vi "flipAndAverageBidirectional.vi"(2 "Depth":dbl[][](graph), 3 "Scan in":refnum<class "Scan.lvclass">) -> (0 "Depth out":dbl[][](graph))   [LabVIEW 2017]
uses:
  classes/Scans/Scan.lvclass
  classes/Scans/Scan.lvclass/Scan.ctl
  classes/Scans/Read A scans.vi
  classes/Scans/Read Total A-scans per frame.vi
  classes/Scans/Read Bidirectional.vi
panel:
  out "size(s) 3":i32[](array[numeric])
  out "size(s) 2":i32[](array[numeric])
  out "size(s)":i32[](array[numeric])
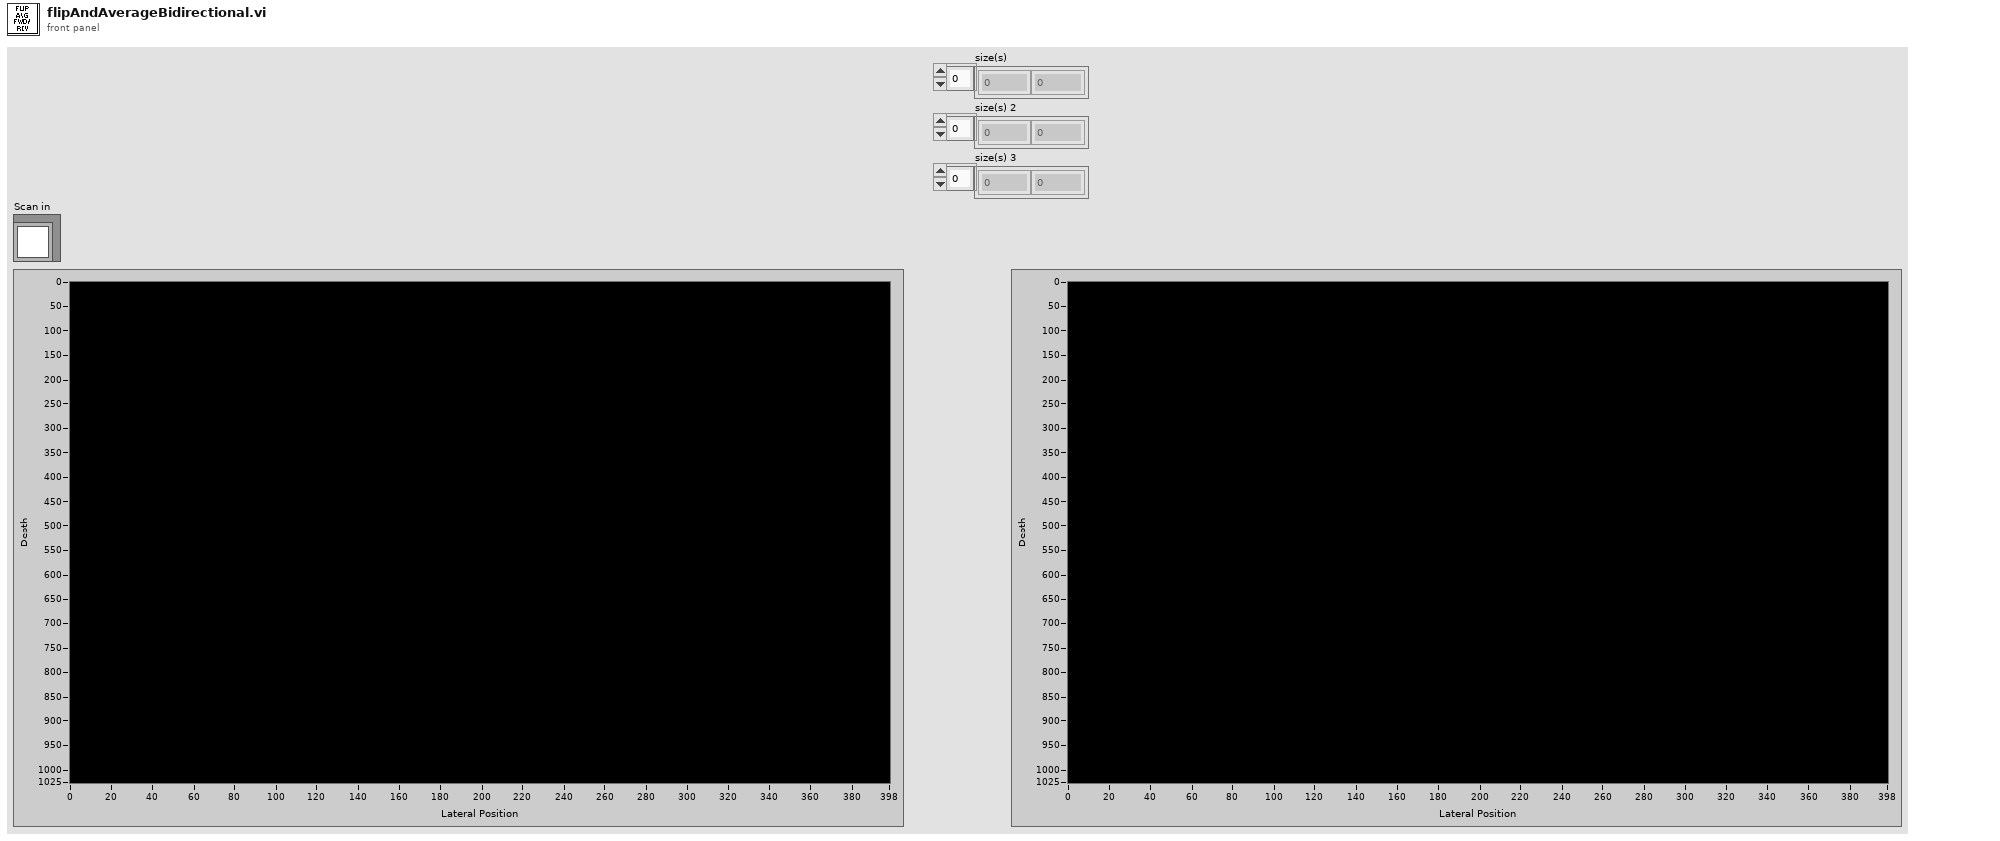
[diagram p1: front panel]
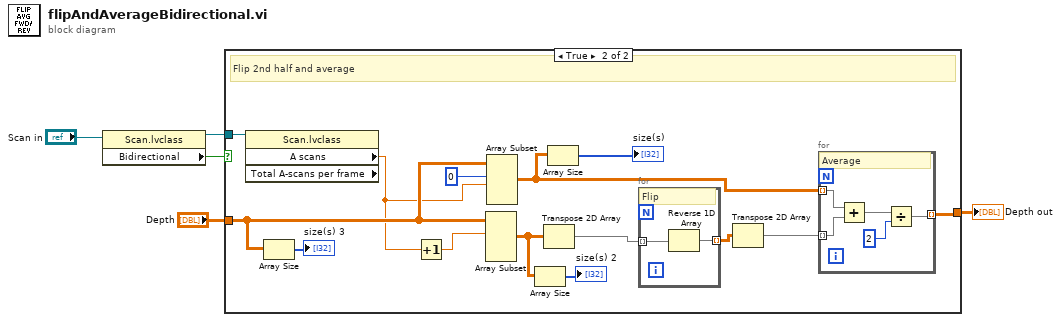
[diagram p0: block diagram]
diagram:
  n1 = property class="Scan.lvclass"(reference="Scan in") -> (reference out=w1:refnum<class "Scan.lvclass">, "Bidirectional"=w4:bool)  [unwired: 1 in, 1 out]
  n2 = case shown="True" w4 {
    tunnel: [w6 w17] -> w2
    tunnel: "Depth" -> [w6 w11]
    tunnel: w1 -> [_ w16]
    frame False {
    }
    frame True {
      # "Flip 2nd half and average"
      n3 = property class="Scan.lvclass" props=["A scans", "Total A-scans per frame"](reference=w16) -> ("A scans"=w8:dbl)  [unwired: 1 in, 3 out]
      n4 = Array Size(array=w11) -> (size(s)=→"size(s) 3":i32[])
      n5 = Increment(x=w8) -> (x+1=w7:dbl)
      n6 = Array Subset(array=w11, index (row)=w7) -> (w13:dbl[][])  [unwired: 3 in]
      n7 = Array Subset(array=w11, index (row)=0 ("index"), length (row)=w8) -> (w15:dbl[][])  [unwired: 2 in]
      n8 = Array Size(array=w13) -> (size(s)=→"size(s) 2":i32[])
      n9 = Transpose 2D Array(2D array=w13) -> (transposed array=w20:dbl[][])
      n10 = Array Size(array=w15) -> (size(s)=→"size(s)":i32[])
      n11 = for {
        tunnel: w20 -> [w27] mode=indexing
        tunnel: [w26] -> w19 mode=indexing
        # "Flip"
        n12 = Reverse 1D Array(array=w27) -> (reversed array=w26:dbl[])
      }
      n13 = Transpose 2D Array(2D array=w19) -> (transposed array=w18:dbl[][])
      n14 = for {
        tunnel: w15 -> [w25] mode=indexing
        tunnel: w18 -> [w24] mode=indexing
        tunnel: [w21] -> w17 mode=indexing
        # "Average"
        n15 = Add(x=w25, y=w24) -> (x+y=w23:dbl[])
        n16 = Divide(x=w23, y=2) -> (x/y=w21:dbl[])
      }
    }
  }
  "Depth out" <- w2
